vi "Pre-Purge Complete.vi"(8 "error in (no error)":errorcluster, 10 "Indicator states in":T2 {"Time Count" format="%.2g"}, 11 "Runtime statuses in":T1) -> (0 "error out":errorcluster, 2 "Indicator states out":T2 {"Time Count" format="%.2g"}, 3 "Runtime statuses out":T1)   [LabVIEW 2014]
doc: "Updates runtime statuses and Boiler indicator states after Pre-Purge is completed"
uses:
  Controls/Boiler Status Indicators.ctl
  Controls/Boiler runtime status indicators.ctl
  Controls/Log file FGV action enum.ctl
  Controls/Log event enum.ctl
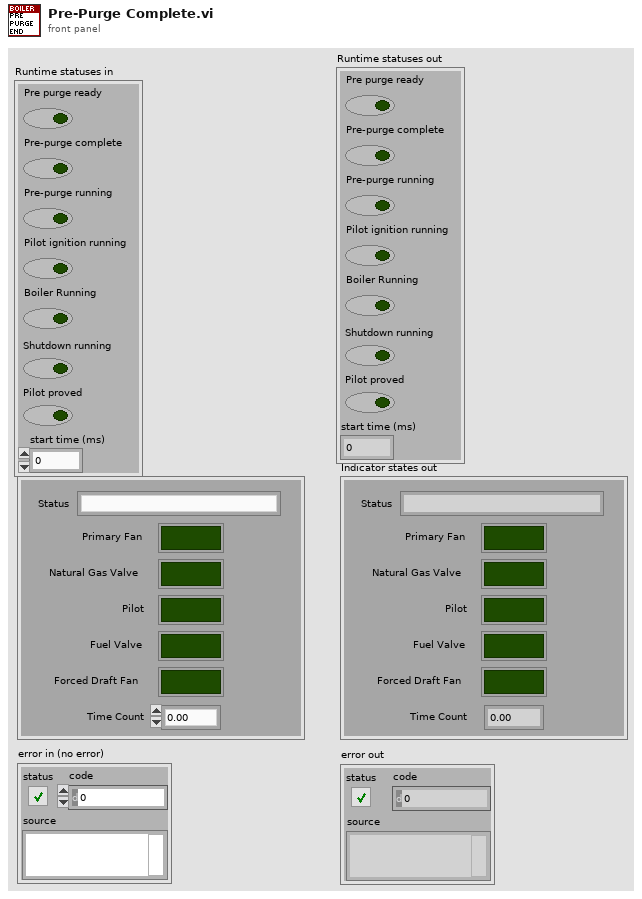
[diagram p1: front panel]
types:
  T1 = typedef "Boiler runtime status indicators.ctl" = cluster{"Pre purge ready":bool, "Pre-purge complete":bool, "Pre-purge running":bool, "Pilot ignition running":bool, "Boiler Running":bool, "Shutdown running":bool, "Pilot proved":bool, "start time (ms)":u32}
  T2 = typedef "Boiler Status Indicators.ctl" = cluster{"Status":string, "Primary Fan":bool, "Natural Gas Valve":bool, "Pilot":bool, "Fuel Valve":bool, "Forced Draft Fan":bool, "Time Count":dbl}
  T3 = typedef "Log event enum.ctl" = enum16{"Boiler Initialized", "Boiler Ready", "Start Pre-Purge", "Pre-Purge Complete", "Pilot ON", "Pilot proved", "Forced Draft Fan ON", "Boiler Running", "Start Shutdown Purge", "Shutdown Purge Complete"}
  T4 = typedef "Log file FGV action enum.ctl" = enum16{"open log file", "log event", "close log file"}
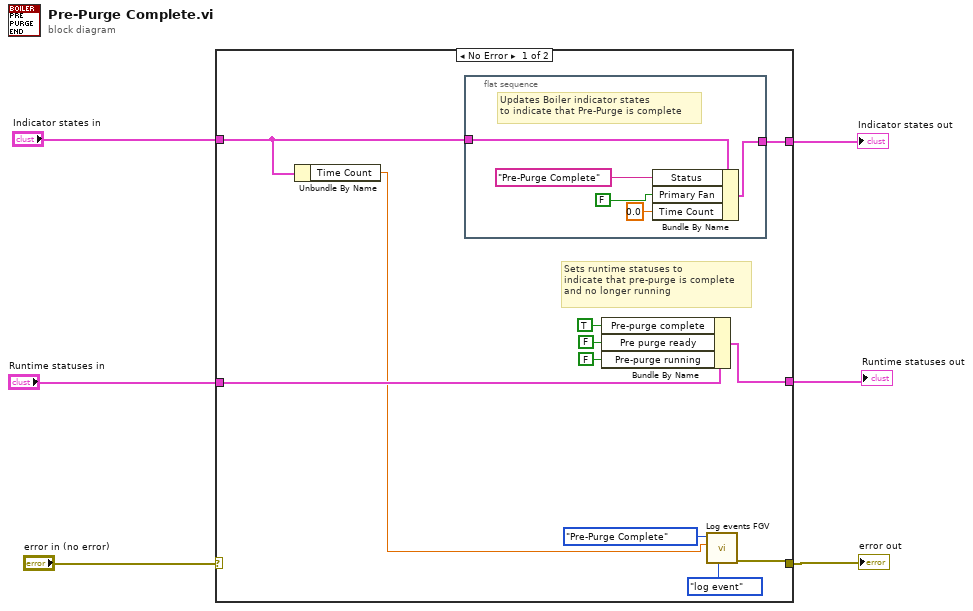
[diagram p0: block diagram]
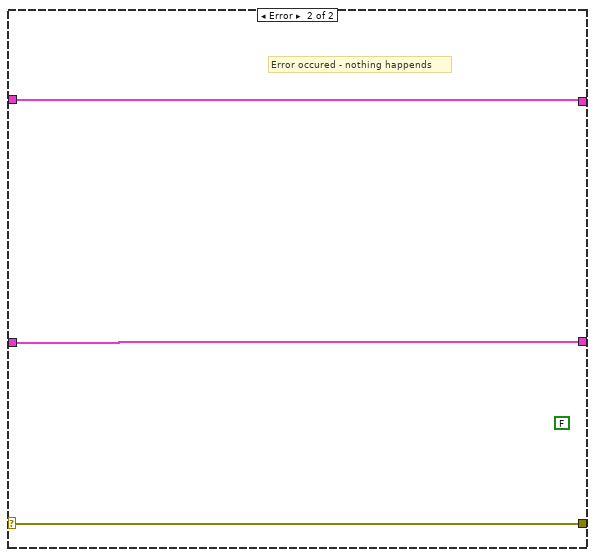
[diagram p2: hidden frame]
diagram:
  n1 = case shown="No Error" "error in (no error)" {
    selector: "error in (no error)" -> [_ w25]
    tunnel: [w9 w25] -> w5
    tunnel: "Runtime statuses in" -> [w16 w23]
    tunnel: "Indicator states in" -> [w8 w24]
    tunnel: [w17 w24] -> w2
    tunnel: [w15 w23] -> w1
    frame No Error {
      # "Sets runtime statuses to\nindicate that pre-purge is complete\nand no longer running"
      n2 = Unbundle By Name(w8) -> ("Time Count"=w7:dbl)
      n3 = flat-sequence {
        tunnel: [w22] -> w17
        tunnel: w8 -> [w18]
        frame #0 {
          # "Updates Boiler indicator states\nto indicate that Pre-Purge is complete"
          n4 = Bundle By Name(cluster=w18, "Status"="Pre-Purge Complete", "Primary Fan"=FALSE, "Time Count"=0.0) -> (w22:T2)
        }
      }
      n5 = Bundle By Name(cluster=w16, "Pre-purge complete"=TRUE, "Pre purge ready"=FALSE, "Pre-purge running"=FALSE ("Pre purge ready")) -> (w15:T1)
      n6 = call "Log events FGV.vi"("action"=Log_file_FGV_action_enum."log event", "Event data"=w7, "Log event"=Log_event_enum."Pre-Purge Complete") -> ("error out"=w9:errorcluster)  [unwired: 8 in]
    }
    frame Error {
      (unwired) FALSE
      # "Error occured - nothing happends"
    }
  }
  "Indicator states out" <- w2
  "error out" <- w5
  "Runtime statuses out" <- w1
